vi "_setControlRef.vi"(7 "parentURL":string, 8 "error in (no error)":errorcluster, 9 "Name":string, 10 "Refnum":refnum<vi>, 11 "TagDB in":T1) -> (0 "error out":errorcluster, 2 "Ref-Key":string, 3 "TagDB out":T1)   [LabVIEW 2017, in "TagDB RefManager.lvlib"]
uses:
  TagDB RefManager.lvlib
  <userlib>/_NEVSTOP/TagDB/Typedef/TagDB.ctl
  39047c58-e22d-481c-91b5-4ba0bd035ec8.vi
  11f946b7-9f57-44fd-b0b0-69ef5a4d0f07.vi
  046b1344-6081-4f7d-b089-6eea8a81863f.vi
  <userlib>/_NEVSTOP/TagDB/_Support/DataAccess/data-Write.vi
  <userlib>/_NEVSTOP/TagDB/_Support/Error/_[error50000]Invalid DB REF.vi
  <userlib>/_NEVSTOP/TagDB/_Support/DataAccess/TagDB Ref to DVR.vi
  <userlib>/_NEVSTOP/TagDB/_Support/DataAccess/_NameCacher.vi
  <userlib>/_NEVSTOP/TagDB/_Support/DataAccess/_datatypeChecker.vi
  <userlib>/_NEVSTOP/TagDB/_Support/Error/_Build Error Cluster.vi
  <vilib>/Utility/Data Type/Get Type Information.vi
  BlackList/_blacklist.vi
  <userlib>/_NEVSTOP/TagDB/TagDB.lvlib
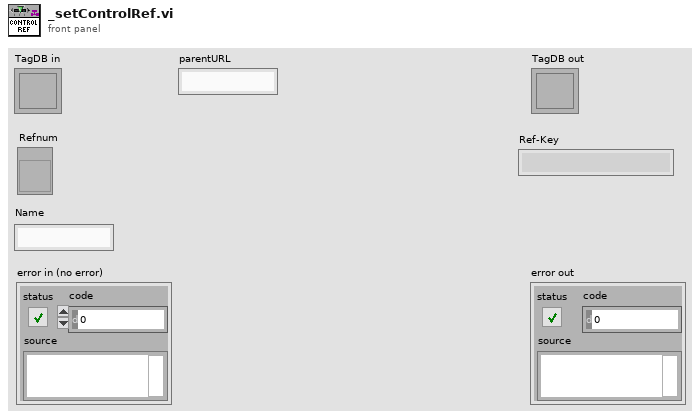
[diagram p1: front panel]
types:
  T1 = typedef "TagDB.lvlib/TagDB.ctl" = refnum<k1>
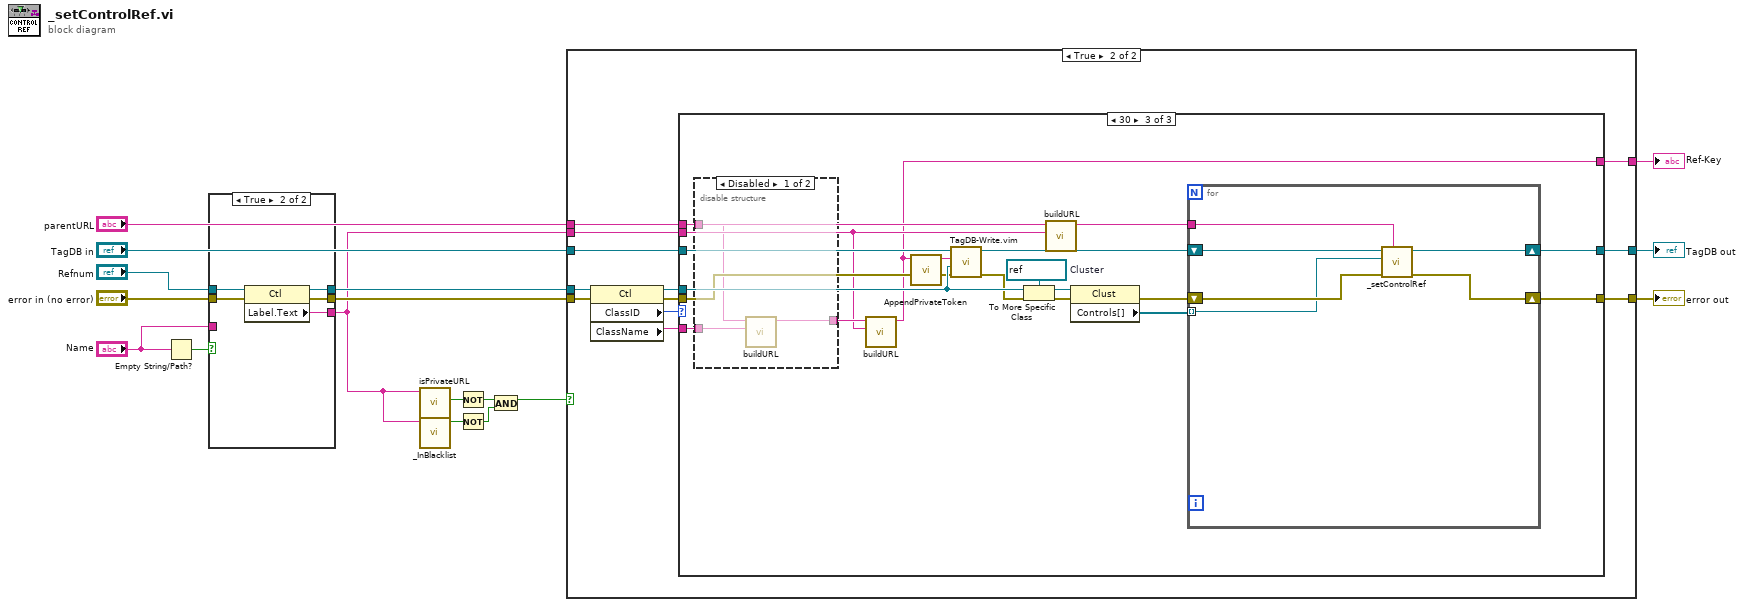
[diagram p0: block diagram]
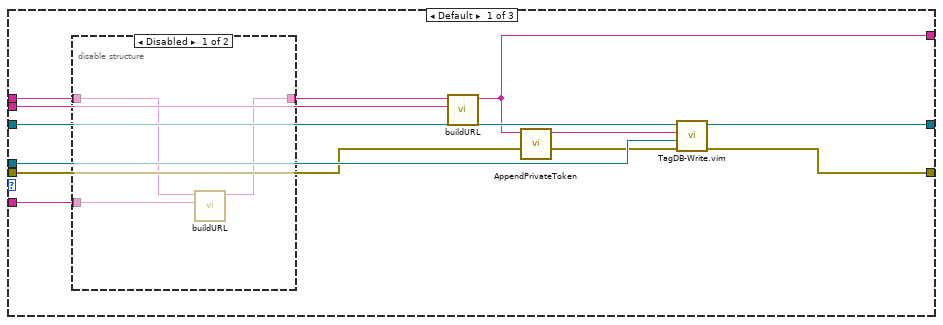
[diagram p3: hidden frame]
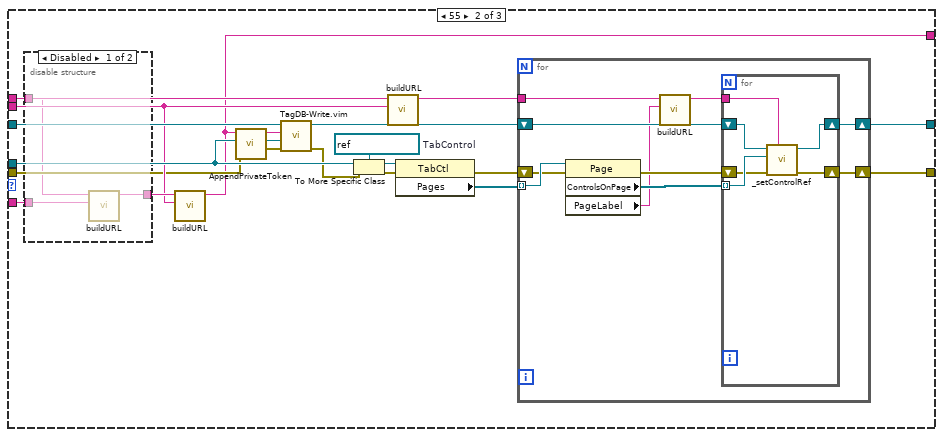
[diagram p5: hidden frame]
diagram:
  n1 = Empty String/Path?(string/path="Name") -> (empty?=w13:bool)
  n2 = case shown="True" w13 {
    tunnel: "error in (no error)" -> [w18 w25]
    tunnel: "Refnum" -> [w19 w24]
    tunnel: [w20 w23] -> w6
    tunnel: [w19 w22] -> w11
    tunnel: [w18 w21] -> w9
    tunnel: "Name" -> [w20 _]
    frame False {
    }
    frame True {
      n3 = property class="Ctl"(reference=w24, error in=w25) -> (reference out=w22:refnum<vi>, error out=w21:errorcluster, "Label.Text"=w23:string)
    }
  }
  n4 = call <userlib>:"isPrivateURL.vi"("URL"=w6) -> ("private?"=w1:bool)  [unwired: 9 in, 1 out]
  n5 = call "_InBlacklist.vi"("String"=w6) -> ("in blacklist?"=w3:bool)  [unwired: 10 in]
  n6 = Not(x=w1) -> (.not. x?=w4:bool)
  n7 = Not(x=w3) -> (.not. x?=w2:bool)
  n8 = And(x=w4, y=w2) -> (x .and. y?=w5:bool)
  n9 = case shown="True" w5 {
    tunnel: "parentURL" -> [w26 w40]
    tunnel: [w27 w36] -> w16
    tunnel: [w28 w35] -> w15
    tunnel: "TagDB in" -> [w28 w34]
    tunnel: w11 -> [_ w33]
    tunnel: w9 -> [w27 w32]
    tunnel: [w26 w31] -> w7
    tunnel: w6 -> [_ w30]
    frame False {
    }
    frame True {
      n10 = property on="Property Node" class="Ctl"(reference=w33, error in=w32) -> (reference out=w37:refnum<vi>, error out=w38:errorcluster, "ClassID"=w39:u32, "ClassName"=w29:string)
      n11 = case shown="30" w39 {
        tunnel: w34 -> [w49 w65 w106]
        tunnel: [w48 w69 w108] -> w35
        tunnel: w38 -> [w43 w60 w104]
        tunnel: [w42 w56 w95] -> w36
        tunnel: w37 -> [w44 w63 w105]
        tunnel: w40 -> [w50 w58 w101]
        tunnel: w30 -> [w47 w61 w99]
        tunnel: [w41 w57 w96] -> w31
        tunnel: w29 -> [w46 w62 w100]
        frame Default {
          n12 = disable-structure shown="Disabled" {
            disable-tunnel: [w54 w55] -> w51
            disable-tunnel: w50 -> [w53 w55]
            disable-tunnel: w46 -> [w52 _]
            frame Disabled {
              n13 = call <userlib>:"buildURL.vi"("DataName"=w52, "parentURL"=w53) -> ("DataURL"=w54:string)  [unwired: 9 in]
            }
            frame Enabled {
            }
          }
          n14 = call <userlib>:"buildURL.vi"("DataName"=w47, "parentURL"=w51) -> ("DataURL"=w41:string)  [unwired: 9 in]
          n15 = call <userlib>:"AppendPrivateToken.vi"("DataURL"=w41) -> ("String"=w45:string)  [unwired: 10 in]
          n16 = call "TagDB-Write.vim"("error in (no error)"=w43, "Value"=w44, "tag"=w45, "TagDB"=w49) -> ("error out"=w42:errorcluster, "TagDB(dup)"=w48:T1)  [unwired: 5 in, 1 out]
        }
        frame 55 {
          w74 = refnum<vi> refnum  # TabControl
          n17 = disable-structure shown="Disabled" {
            disable-tunnel: [w77 w78] -> w67
            disable-tunnel: w62 -> [w76 _]
            disable-tunnel: w58 -> [w75 w78]
            frame Disabled {
              n18 = call <userlib>:"buildURL.vi"("DataName"=w76, "parentURL"=w75) -> ("DataURL"=w77:string)  [unwired: 9 in]
            }
            frame Enabled {
            }
          }
          n19 = call <userlib>:"buildURL.vi"("DataName"=w61, "parentURL"=w67) -> ("DataURL"=w57:string)  [unwired: 9 in]
          n20 = call <userlib>:"AppendPrivateToken.vi"("DataURL"=w57) -> ("String"=w66:string)  [unwired: 10 in]
          n21 = call "TagDB-Write.vim"("error in (no error)"=w60, "Value"=w63, "tag"=w66, "TagDB"=w65) -> ("error out"=w59:errorcluster, "TagDB(dup)"=w64:T1)  [unwired: 5 in, 1 out]
          n22 = To More Specific Class(target class=w74, reference=w63, error in=w59) -> (specific class reference=w73:refnum<vi>, error out=w72:errorcluster)
          n23 = call <userlib>:"buildURL.vi"("DataName"=w61, "parentURL"=w58) -> ("DataURL"=w68:string)  [unwired: 9 in]
          n24 = property class="TabCtl"(reference=w73, error in=w72) -> (error out=w70:errorcluster, "Pages"=w71:refnum<vi>[])  [unwired: 1 out]
          n25 = for {
            tunnel: w71 -> [w88] mode=indexing
            shift-right: [w82] -> w56
            shift-left: w70 -> [w87]
            shift-right: [w84] -> w69
            shift-left: w64 -> [w85]
            tunnel: w68 -> [w80]
            n26 = property class="Page"(reference=w88, error in=w87) -> (error out=w83:errorcluster, "ControlsOnPage"=w86:refnum<vi>[], "PageLabel"=w79:string)  [unwired: 1 out]
            n27 = call <userlib>:"buildURL.vi"("DataName"=w79, "parentURL"=w80) -> ("DataURL"=w81:string)  [unwired: 9 in]
            n28 = for {
              tunnel: w86 -> [w94] mode=indexing
              shift-right: [w92] -> w84
              shift-left: w85 -> [w93]
              shift-right: [w90] -> w82
              shift-left: w83 -> [w91]
              tunnel: w81 -> [w89]
              n29 = call "_setControlRef.vi"("parentURL"=w89, "error in (no error)"=w91, "Refnum"=w94, "TagDB in"=w93) -> ("error out"=w90:errorcluster, "TagDB out"=w92:T1)  [unwired: 5 in, 1 out]
            }
          }
        }
        frame 30 {
          w113 = refnum<vi> refnum  # Cluster
          n30 = disable-structure shown="Disabled" {
            disable-tunnel: [w116 w117] -> w102
            disable-tunnel: w101 -> [w115 w117]
            disable-tunnel: w100 -> [w114 _]
            frame Disabled {
              n31 = call <userlib>:"buildURL.vi"("DataName"=w114, "parentURL"=w115) -> ("DataURL"=w116:string)  [unwired: 9 in]
            }
            frame Enabled {
            }
          }
          n32 = call <userlib>:"buildURL.vi"("DataName"=w99, "parentURL"=w102) -> ("DataURL"=w96:string)  [unwired: 9 in]
          n33 = call <userlib>:"AppendPrivateToken.vi"("DataURL"=w96) -> ("String"=w98:string)  [unwired: 10 in]
          n34 = call "TagDB-Write.vim"("error in (no error)"=w104, "Value"=w105, "tag"=w98, "TagDB"=w106) -> ("error out"=w103:errorcluster, "TagDB(dup)"=w97:T1)  [unwired: 5 in, 1 out]
          n35 = To More Specific Class(target class=w113, reference=w105, error in=w103) -> (specific class reference=w112:refnum<vi>, error out=w111:errorcluster)
          n36 = call <userlib>:"buildURL.vi"("DataName"=w99, "parentURL"=w101) -> ("DataURL"=w107:string)  [unwired: 9 in]
          n37 = property class="Clust"(reference=w112, error in=w111) -> (error out=w109:errorcluster, "Controls[]"=w110:refnum<vi>[])  [unwired: 1 out]
          n38 = for {
            tunnel: w110 -> [w118] mode=indexing
            shift-right: [w121] -> w95
            shift-left: w109 -> [w119]
            shift-right: [w122] -> w108
            shift-left: w97 -> [w123]
            tunnel: w107 -> [w120]
            n39 = call "_setControlRef.vi"("parentURL"=w120, "error in (no error)"=w119, "Refnum"=w118, "TagDB in"=w123) -> ("error out"=w121:errorcluster, "TagDB out"=w122:T1)  [unwired: 5 in, 1 out]
          }
        }
      }
    }
  }
  "error out" <- w16
  "TagDB out" <- w15
  "Ref-Key" <- w7
